vi "DSF.Engine.Memory.Cache.Framework.Get Plugin Caches.vi"(8 "error in (no error)":errorcluster, 11 "Framework Cache in":refnum<class "DSF.Engine.Memory.Cache.Framework.lvclass">) -> (0 "error out":errorcluster, 2 "Plugin Caches":refnum<class "DSF.Engine.Memory.Cache.Plugin.lvclass">[](array[class]), 3 "Framework Cache out":refnum<class "DSF.Engine.Memory.Cache.Framework.lvclass">)   [LabVIEW 2016, in "DSF.Engine.lvlib" / "DSF.Engine.Memory.Cache.Framework.lvclass"]
uses:
  Cache/DSF.Engine.Memory.Cache.Framework.lvclass
  DSF.Engine.Memory.Cache.Plugin.lvclass
  Cache/DSF.Engine.Memory.Cache.Framework.lvclass/DSF.Engine.Memory.Cache.Framework.ctl
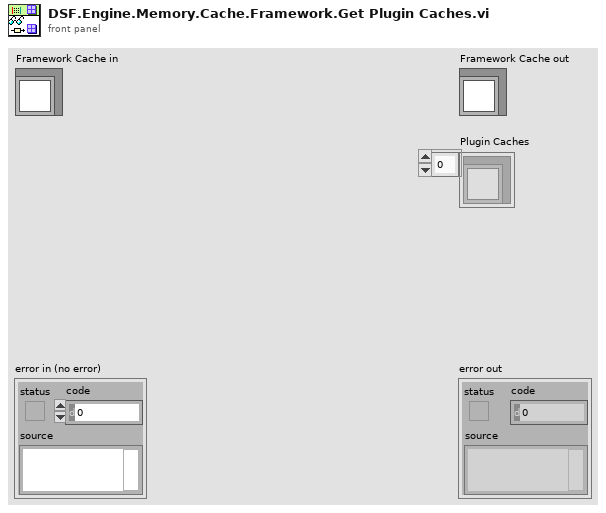
[diagram p1: front panel]
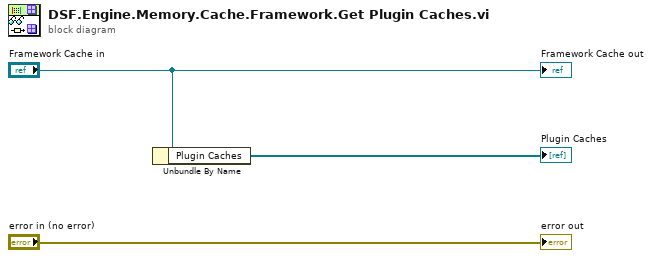
[diagram p0: block diagram]
diagram:
  n1 = Unbundle By Name("Framework Cache in") -> ("Plugin Caches"=→"Plugin Caches":refnum<class "DSF.Engine.Memory.Cache.Plugin.lvclass">[])
  "error out" <- "error in (no error)"
  "Framework Cache out" <- "Framework Cache in"
